vi "Event Nested Status.vi"(11 "Hello World Queue in":refnum<class "Hello World Queue.lvclass">) -> (0 "Event Nested Count":i32, 1 "Event Nested Aliases":string[](array[string]), 2 "Any Exist?":bool, 3 "Hello World Queue out":refnum<class "Hello World Queue.lvclass">)   [LabVIEW 2021, in "Hello World Queue.lvlib" / "Hello World Queue.lvclass"]
uses:
  Hello World Queue.lvclass
  Hello World Queue.lvclass/Hello World Queue.ctl
  jettl/Queue jettl/Queue jettl.lvclass
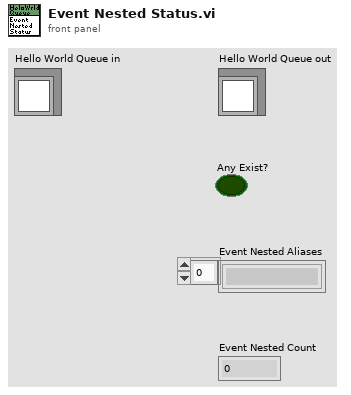
[diagram p1: front panel]
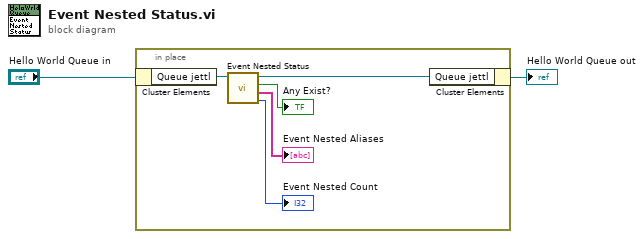
[diagram p0: block diagram]
diagram:
  n1 = in-place {
    n2 = in-place-cluster #1("Hello World Queue in") -> ("Queue jettl"=w4:refnum<class "Queue jettl.lvclass">)
    n3 = call-dynamic "Event Nested Status.vi"("Queue jettl in"=w4) -> ("Event Nested Count"=→"Event Nested Count":i32, "Event Nested Aliases"=→"Event Nested Aliases":string[], "Any Exist?"=→"Any Exist?":bool, "Queue jettl out"=w3:refnum<class "Queue jettl.lvclass">)  [unwired: 7 in]
    n4 = in-place-cluster #1("Queue jettl"=w3) -> (→"Hello World Queue out":refnum<class "Hello World Queue.lvclass">)
  }
